vi "Open.vi"   [LabVIEW 2023, in "SQLite.lvlib" / "Connection.lvclass"]
doc: "Opens (or creates) an SQLite3 database file, using a supplied filename as a path or a string (On a Mac, the string must be in Unix format, e.g. \"/Users/.../filename.db\").\n\nSupplying the string \":memory:\" causes an in-memory database to be created, while supplying an empty string causes a temporary database to be created. Both of these are destroyed when the connection is closed.\n\nBusy timeout is the time opertions such as \"Step\" will wait when the database is locked by another connection before returning an error. Default is 5000 ms. \n\nAn alternate SQLite3 shared library may be specified, otherwise the default one included with the package will be used. On Macs, this is the default version of SQLite3 include with the OSX operating system.\n\nThe optional connection for \"SQLite Connection type\" is intended for use with child classes of \"SQLite Connection\"."
uses:
  Connection.lvclass
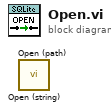
[diagram p0: block diagram]
diagram:
  n1 = call "Open (string).vi"() -> ()  [unwired: 10 in, 2 out]
  n2 = call "Open (path).vi"() -> ()  [unwired: 10 in, 2 out]
